vi "浊度电极校准.vi"() -> ()   [LabVIEW 2016, in "斯坦道多参数.lvlib"]
uses:
  <vilib>/Utility/miscctls.llb/LVPointTypeDef.ctl
  <vilib>/Utility/miscctls.llb/LVPositionTypeDef.ctl
  <vilib>/Analysis/NI_AALBase.lvlib
panel:
  out "温度":dbl format="%#.2f"
  out "通讯状态":string
  out "电极状态标志":u16(ring) items=["OK"=0, "第一点校正通过"=1, "第二点校正通过"=2, "悬浮物两点校准第一点校正通过"=11, "悬浮物两点校准第二点校正通过"=12, "浊度三点校正第一点校正通过"=31, "浊度三点校正第二点校正通过"=32, "浊度三点校正第三点校正通过"=33]
  out "第三点校准值":dbl
  out "标液3":dbl
  out "第二点校准值":dbl
  out "第一点校准值":dbl
  in  "校准停止":bool
  in  "校准启动":bool
  in  "校准模式":enum16{"两点校准", "单点校准", "三点校准"}(ring)
  out "最小值":sgl format="%#.2f"
  out "最大值":sgl format="%#.2f"
  out "波形图表":sgl(graph) caption="历史曲线"
  out "mean":dbl caption="均值" format="%#.2f"
  out "standard deviation":dbl caption="标准差" format="%#.2f"
  out "变异系数":dbl format="%#.6f"
  out "测量值":dbl format="%#.2f"
  out "提示":string
  out "标液2":dbl
  out "标液1":dbl
  out "原始读取值":dbl caption="信号值" format="%#.2f"
  out "偏移值补偿":dbl format="%#.2f"
  out "电极斜率":dbl format="%#.6f"
  out "电极零点":dbl format="%#.6f"
  # "浊度电极设定"
  # "℃"
  # "NTU"
  # "%"
  # "NTU"
  # "请选择校准模式:"
  # "NTU"
  # "NTU"
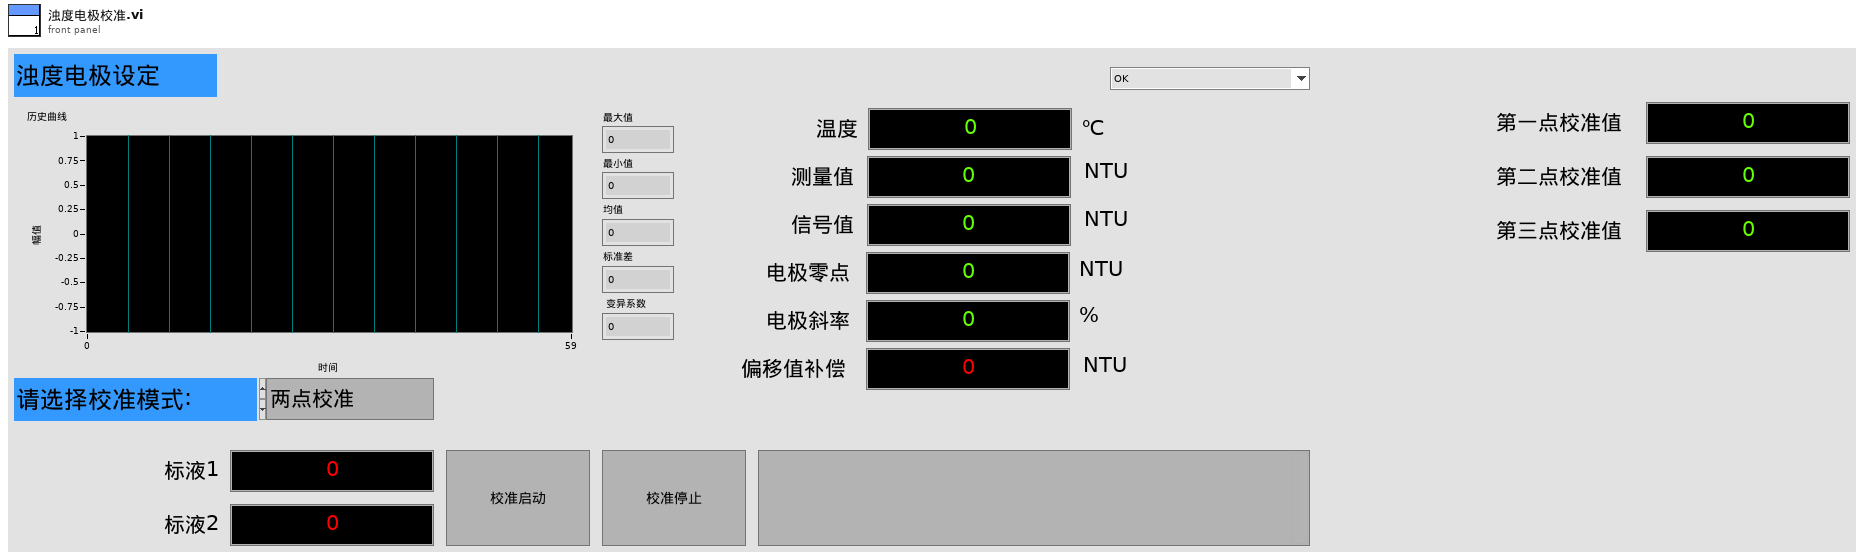
[diagram p1: front panel]
types:
  T1 = typedef "LVPointTypeDef.ctl" = cluster{"Horizontal":i16, "Vertical":i16}
  T2 = typedef "斯坦道多参数.lvlib/校准步骤.ctl" = enum16{"待机", "放置第一点标液", "第一点校准启动", "第一点校准写入", "第一点校准失败", "放置第二点标液", "第二点校准启动", "第二点校准写入", "第二点校准失败", "放置第三点标液", "第三点校准启动", "第三点校准写入", "第三点校准失败", "校准结果写入", "校准结束"}
  T3 = cluster{"电极状态标志":u16, "电极型号标志":u16, "浊度测量值":sgl, "温度测量值":sgl, "浊度信号值":sgl, "浊度偏移修正值":sgl, "温度偏移修正值":sgl, "手动温度补偿值":sgl, "浊度电极零点":sgl, "浊度电极斜率":sgl, "第1点标准值记录":sgl, "第1点信号值记录":sgl, "第1点温度值记录":sgl, "第2点标准值记录":sgl, "第2点信号值记录":sgl, "第2点温度值记录":sgl, "命令滤波设定":u16, "温度模式":enum16{"ATC", "MTC"}, "生产批次":u16, "电极序号":u16, "串口地址":u16, "串口波特率":enum16{"9600", "19200", "115200"}, "串口校验位":enum16{"NONE", "ODD", "EVEN"}, "串口停止位":enum16{"1bit", "2bit"}, "第一点标准值":sgl, "第二点标准值":sgl, "第三点标准值":sgl}
  T4 = typedef "LVPositionTypeDef.ctl" = cluster{"Left":i32, "Top":i32}
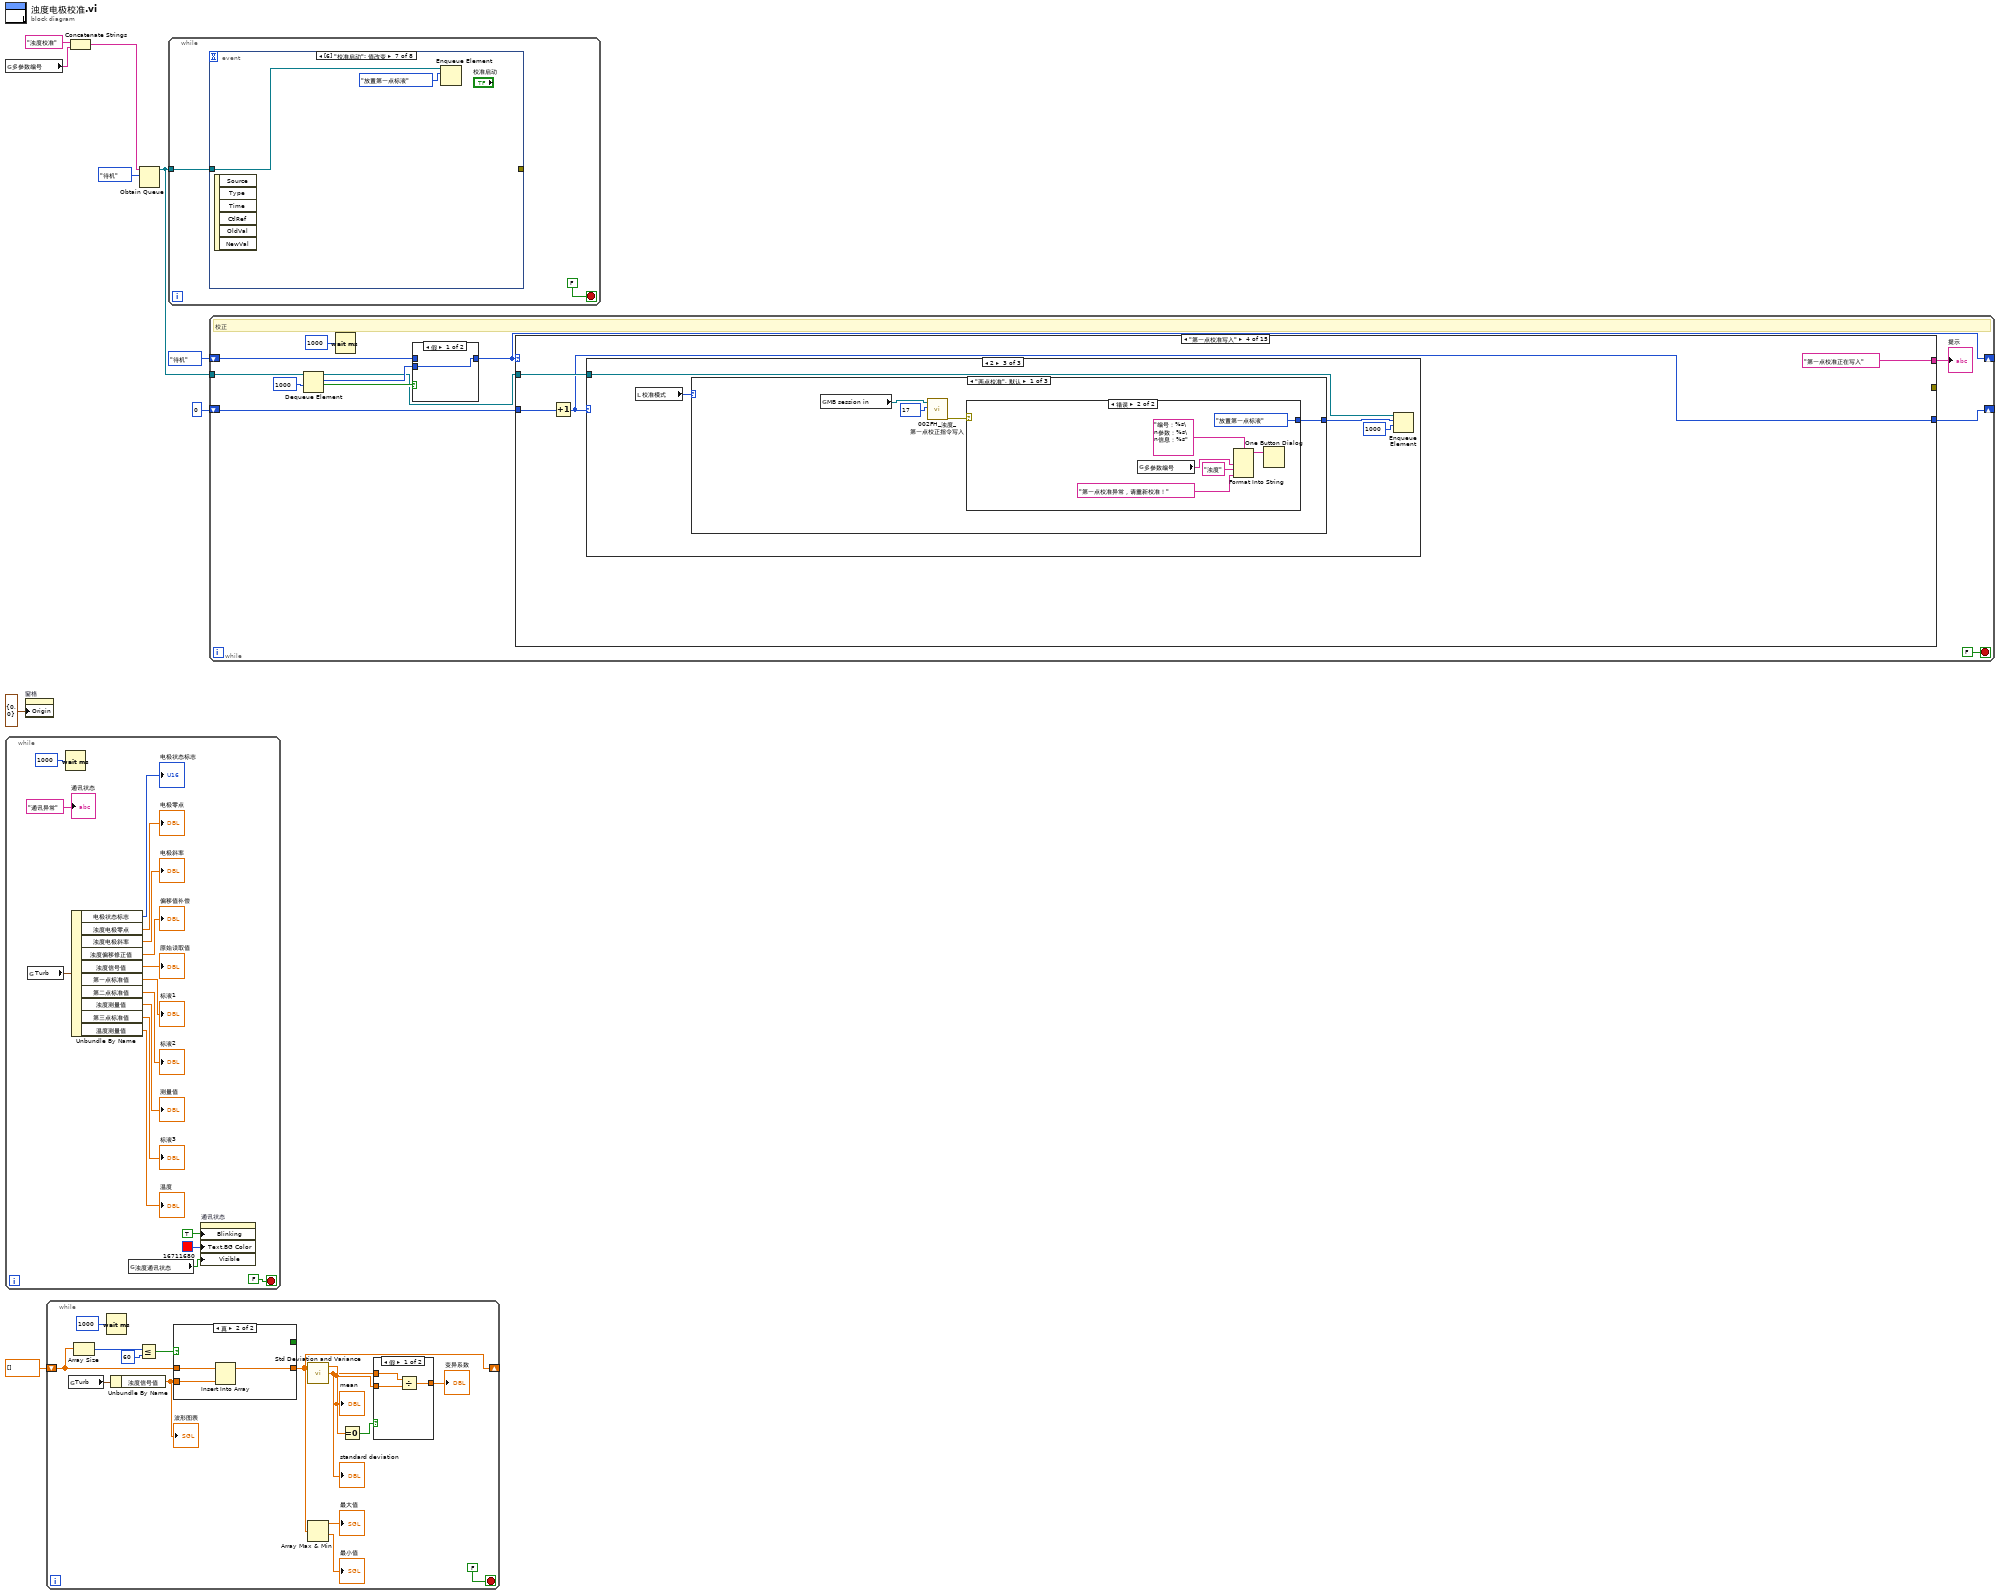
[diagram p0: block diagram]
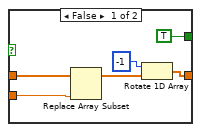
[diagram p3: hidden frame]
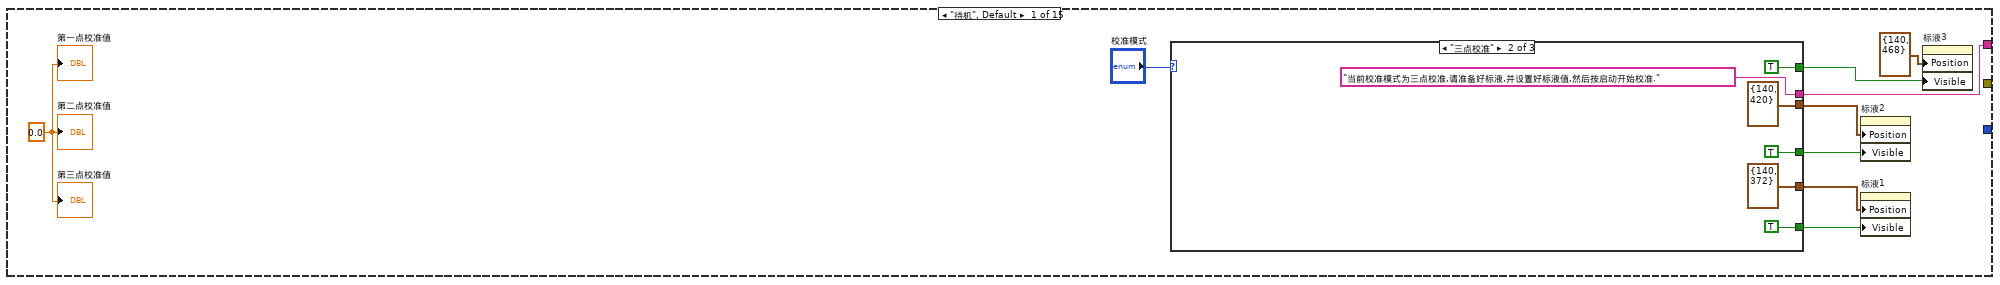
[diagram p5: hidden frame]
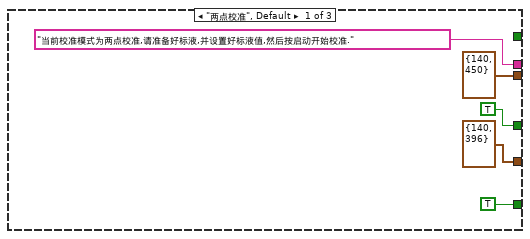
[diagram p6: hidden frame]
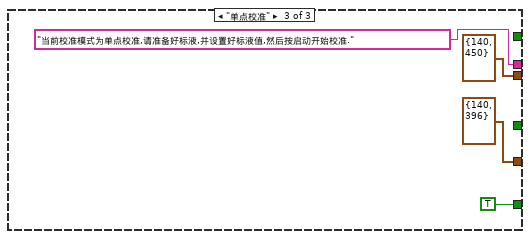
[diagram p7: hidden frame]
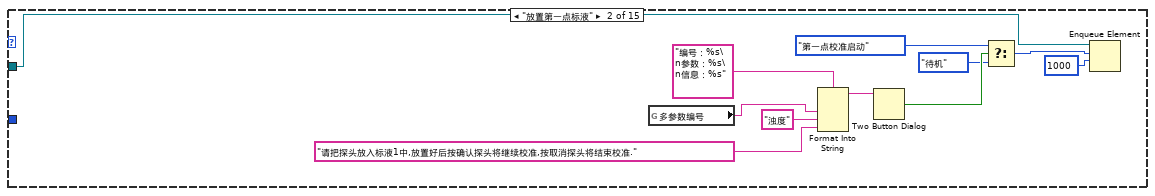
[diagram p8: hidden frame]
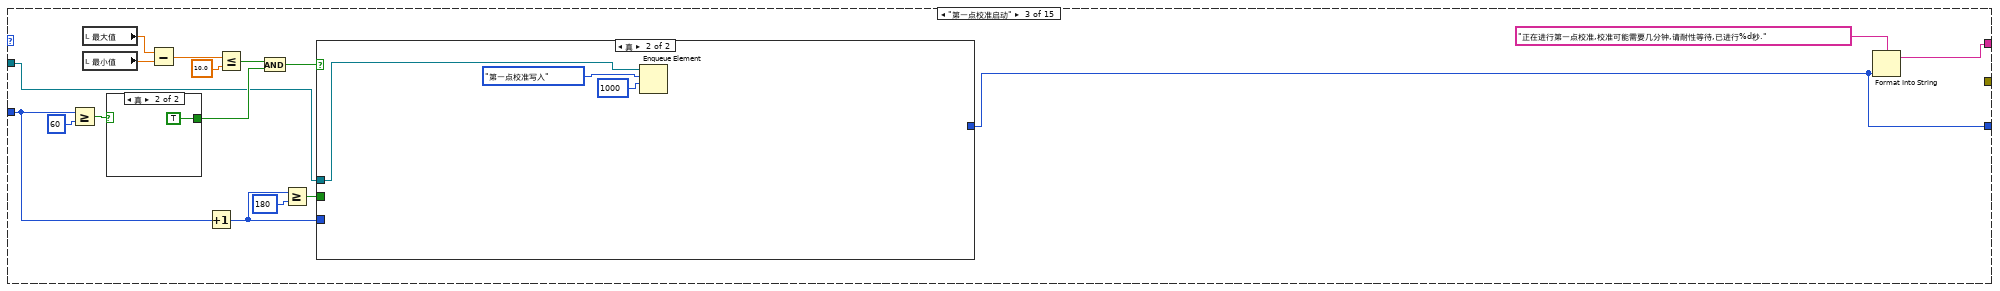
[diagram p9: hidden frame]
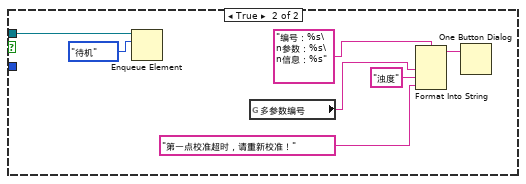
[diagram p11: hidden frame]
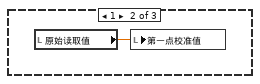
[diagram p14: hidden frame]
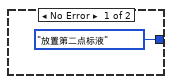
[diagram p15: hidden frame]
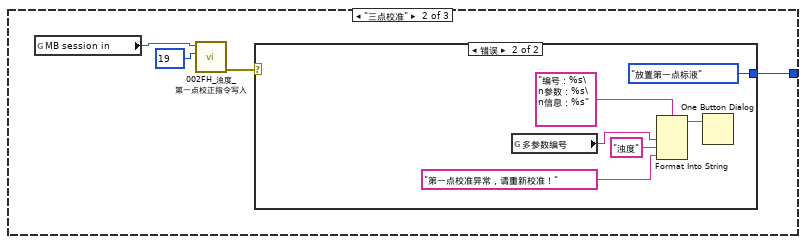
[diagram p16: hidden frame]
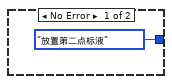
[diagram p17: hidden frame]
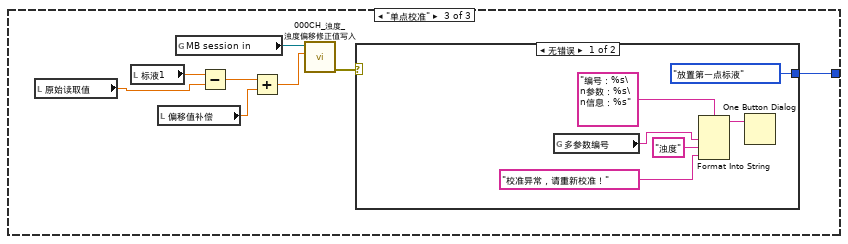
[diagram p18: hidden frame]
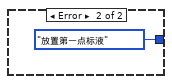
[diagram p19: hidden frame]
diagram:
  n1 = global read "多参数全局变量.vi" "多参数编号"() -> (w1:string)
  n2 = while {
    stop <- FALSE stop-if-true
    n3 = global read "国弘过程全局变量.vi" "Turb"() -> (w24:T3)
    n4 = Wait (ms)(milliseconds to wait=u32 1000 ("等待时间（毫秒）")) -> ()  [unwired: 1 out]
    n5 = Unbundle By Name(w24) -> ("电极状态标志"=→"电极状态标志":u16, "浊度电极零点"=→"电极零点":sgl, "浊度电极斜率"=→"电极斜率":sgl, "浊度偏移修正值"=→"偏移值补偿":sgl, "浊度信号值"=→"原始读取值":sgl, "第一点标准值"=→"标液1":sgl, "第二点标准值"=→"标液2":sgl, "浊度测量值"=→"测量值":sgl, "第三点标准值"=→"标液3":sgl, "温度测量值"=→"温度":sgl)
    n6 = global read "多参数全局变量.vi" "浊度通讯状态"() -> (w12:bool)
    n7 = property on="通讯状态" class="Str"("Blinking"=TRUE ("闪烁"), "Text.BG Color"=u32 16711680, "Visible"=w12) -> ()  [unwired: 2 in, 2 out]
    "通讯状态" <- "通讯异常" ("当前串口")
  }
  n8 = property on="窗格" class="Pane"("Origin"=T1 {"Horizontal"=0, "Vertical"=0} ("原点")) -> ()  [unwired: 2 in, 2 out]
  n9 = while {
    shift-right: [w30] -> _
    shift-left: sgl[] [] -> [w37]
    stop <- FALSE stop-if-true
    n10 = global read "国弘过程全局变量.vi" "Turb"() -> (w31:T3)
    n11 = Array Size(array=w37) -> (size(s)=w39:i32)
    n12 = Wait (ms)(milliseconds to wait=u32 1000 ("等待时间（毫秒）")) -> ()  [unwired: 1 out]
    n13 = Unbundle By Name(w31) -> ("浊度信号值"=w27:sgl)
    "波形图表" <- w27
    n14 = Less Or Equal?(x=w39, y=60) -> (x <= y?=w38:bool)
    n15 = case shown="真" w38 {
      tunnel: w37 -> [w50 w53]
      tunnel: w27 -> [w48 w52]
      tunnel: [w46 w51] -> w30
      tunnel: [TRUE _] -> _
      frame False {
        n16 = Replace Array Subset(array=w50, new element=w48) -> (w49:sgl[])  [unwired: 1 in]
        n17 = Rotate 1D Array(1:w49, 2:-1 ("n")) -> (0:w46:sgl[])
      }
      frame True {
        n18 = Insert Into Array(array=w53, new element=w52) -> (w51:sgl[])  [unwired: 1 in]
      }
    }
    n19 = call <vilib>:"Std Deviation and Variance.vi"("X"=w30) -> ("mean"=w35:dbl, "standard deviation"=w34:dbl)  [unwired: 1 in, 1 out]
    "mean" <- w35
    "standard deviation" <- w34
    n20 = Array Max & Min(array=w30) -> (max value=→"最大值":sgl, min value=→"最小值":sgl)  [unwired: 2 out]
    n21 = Equal To 0?(x=w35) -> (x = 0?=w36:bool)
    n22 = case shown="假" w36 {
      tunnel: w34 -> [w44 _]
      tunnel: [w43 _] -> w33
      tunnel: w35 -> [w42 _]
      frame False {
        n23 = Divide(x=w44, y=w42) -> (x/y=w43:dbl)
      }
      frame True {
      }
    }
    "变异系数" <- w33
  }
  n24 = Concatenate Strings("浊度校准" ("名称（未命名）"), w1) -> (w2:string)
  n25 = Obtain Queue(name (unnamed)=w2, element data type=校准步骤."待机" ("枚举")) -> (queue out=w4:refnum<queue>)  [unwired: 3 in, 2 out]
  n26 = while {
    tunnel: w4 -> [w54]
    stop <- FALSE stop-if-true
    n27 = event shown="[6] \"校准启动\": 值改变" {
      selector: _ -> [_ _ _ _ _ _ _ _]
      dyn-events: _ -> [_ _ _ _ _ _ _ _]
      timeout: _ -> [_ _ _ _ _ _ _ _]
      tunnel: [_ _ w61 w64 w68 w71 _ _] -> _
      tunnel: w54 -> [_ _ _ _ _ _ w72 w74]
      event Timeout {
        n28 = event-data() -> ()  [unwired: 1 in, 3 out]
      }
      event "偏移值补偿", "标液1", "标液2", "标液3": Mouse Down {
        n29 = event-data() -> ("CtlRef"=w56:refnum<vi>)  [unwired: 1 in, 7 out]
        n30 = property class="DigNum (严格)"(reference=w56) -> (reference out=w57:refnum<vi>, "Value"=w58:dbl)  [unwired: 1 in, 1 out]
        n31 = call "数字键盘.vi"("OldNumber"=w58) -> ("NewNumber"=w59:dbl)  [unwired: 1 in]
        n32 = property class="DigNum (严格)"(reference=w57, "Val(Sgnl)"=w59) -> ()  [unwired: 1 in, 2 out]
      }
      event "偏移值补偿": Value Change {
        n33 = event-data() -> ("NewVal"=w62:dbl)  [unwired: 1 in, 5 out]
        n34 = global read "多参数全局变量.vi" "MB session in"() -> (w60:refnum<class "MB_Master.lvclass">)
        n35 = call "000CH_浊度_浊度偏移修正值写入.vi"("数值"=w62, "MB session in"=w60) -> ("error out"=w61:errorcluster)  [unwired: 8 in, 1 out]
      }
      event "标液1": Value Change {
        n36 = event-data() -> ("NewVal"=w65:dbl)  [unwired: 1 in, 5 out]
        n37 = global read "多参数全局变量.vi" "MB session in"() -> (w63:refnum<class "MB_Master.lvclass">)
        n38 = call "0030H_浊度_第一点标准值写入.vi"("数值"=w65, "MB session in"=w63) -> ("error out"=w64:errorcluster)  [unwired: 8 in, 1 out]
      }
      event "标液2": Value Change {
        n39 = event-data() -> ("NewVal"=w67:dbl)  [unwired: 1 in, 5 out]
        n40 = global read "多参数全局变量.vi" "MB session in"() -> (w66:refnum<class "MB_Master.lvclass">)
        n41 = call "0033H_浊度_第二点标准值写入.vi"("数值"=w67, "MB session in"=w66) -> ("error out"=w68:errorcluster)  [unwired: 8 in, 1 out]
      }
      event "标液3": Value Change {
        n42 = event-data() -> ("NewVal"=w70:dbl)  [unwired: 1 in, 5 out]
        n43 = global read "多参数全局变量.vi" "MB session in"() -> (w69:refnum<class "MB_Master.lvclass">)
        n44 = call "0036H_浊度_第三点标准值写入.vi"("数值"=w70, "MB session in"=w69) -> ("error out"=w71:errorcluster)  [unwired: 8 in, 1 out]
      }
      event "校准启动": Value Change {
        n45 = event-data() -> ()  [unwired: 1 in, 6 out]
        n46 = Enqueue Element(queue=w72, element=校准步骤."放置第一点标液" ("元素")) -> ()  [unwired: 2 in, 3 out]
      }
      event "校准停止": Value Change {
        n47 = event-data() -> ()  [unwired: 1 in, 6 out]
        n48 = Flush Queue(queue=w74) -> (queue out=w75:refnum<queue>)  [unwired: 1 in, 2 out]
        n49 = Enqueue Element(queue=w75, element=校准步骤."待机" ("元素"), timeout in ms (-1)=1000 ("超时毫秒(-1)")) -> ()  [unwired: 1 in, 3 out]
      }
    }
  }
  n50 = while "While循环" {
    shift-right: [w79] -> _
    shift-left: 校准步骤."待机" ("枚举") -> [w81]
    shift-right: [w78] -> _
    shift-left: 0 -> [w87]
    tunnel: w4 -> [w82]
    stop <- FALSE stop-if-true
    # "校正"
    n51 = Dequeue Element(queue=w82, timeout in ms (-1)=1000 ("超时毫秒(-1)")) -> (queue out=w80:refnum<queue>, element=w83:T2, timed out?=w84:bool)  [unwired: 1 in, 1 out]
    n52 = Wait (ms)(milliseconds to wait=u32 1000 ("等待时间（毫秒）")) -> ()  [unwired: 1 out]
    n53 = case shown="假" w84 {
      tunnel: w83 -> [w90 _]
      tunnel: [w90 w91] -> w79
      tunnel: w81 -> [_ w91]
      frame False {
      }
      frame True {
      }
    }
    n54 = case shown="\"第一点校准写入\"" w79 {
      tunnel: [w99 _ w128 "第一点校准正在写入" ("提示") _ _ w219 "第二点校准正在写入" ("提示") "第二点校准失败" ("提示") _ "第三点校准正在写入" ("提示") w315 "第三点校准失败" ("提示") w349 w384] -> w86
      tunnel: w87 -> [_ _ w129 w162 _ _ w220 w252 _ _ w297 w316 _ _ _]
      tunnel: [_ _ w127 w160 _ _ w218 w250 _ _ w295 w314 _ _ _] -> w78
      tunnel: w80 -> [_ w121 w130 w161 _ w211 w221 w251 _ w289 w296 w317 _ w355 _]
      tunnel: [_ _ _ _ _ _ _ _ _ _ _ _ _ w354 _] -> _
      frame "待机", Default {
        w92 = 0.0 ("第一点校准值")
        n55 = case shown="\"三点校准\"" "校准模式" {
          tunnel: ["当前校准模式为两点校准,请准备好标液,并设置好标液值,然后按启动开始校准." ("提示") "当前校准模式为三点校准,请准备好标液,并设置好标液值,然后按启动开始校准." ("提示") "当前校准模式为单点校准,请准备好标液,并设置好标液值,然后按启动开始校准." ("提示")] -> w99
          tunnel: [TRUE ("可见") TRUE ("可见") _] -> w95
          tunnel: [T4 {"Left"=140, "Top"=396} ("位置") T4 {"Left"=140, "Top"=372} ("位置") T4 {"Left"=140, "Top"=396} ("位置")] -> w98
          tunnel: [T4 {"Left"=140, "Top"=450} ("位置 2") T4 {"Left"=140, "Top"=420} ("位置 2") T4 {"Left"=140, "Top"=450} ("位置 2")] -> w97
          tunnel: [_ TRUE ("可见") _] -> w94
          tunnel: [TRUE ("可见") TRUE ("可见") TRUE ("可见")] -> w93
          frame "两点校准", Default {
          }
          frame "三点校准" {
          }
          frame "单点校准" {
          }
        }
        n56 = property on="标液2" class="DigNum (严格)"("Position"=w97, "Visible"=w95) -> ()  [unwired: 2 in, 2 out]
        n57 = property on="标液1" class="DigNum (严格)"("Position"=w98, "Visible"=w93) -> ()  [unwired: 2 in, 2 out]
        n58 = property on="标液3" class="DigNum (严格)"("Position"=T4 {"Left"=140, "Top"=468} ("位置 3"), "Visible"=w94) -> ()  [unwired: 2 in, 2 out]
        "第一点校准值" <- w92
        "第二点校准值" <- w92
        "第三点校准值" <- w92
      }
      frame "放置第一点标液" {
        n59 = global read "多参数全局变量.vi" "多参数编号"() -> (w119:string)
        n60 = Format Into String(format string="编号：%s\n参数：%s\n信息：%s" ("格式字符串"), w119, "浊度" ("输入 2"), "请把探头放入标液1中,放置好后按确认探头将继续校准,按取消探头将结束校准." ("消息")) -> (resulting string=w116:string)  [unwired: 2 in, 1 out]
        n61 = Two Button Dialog(message=w116) -> (T button?=w125:bool)  [unwired: 2 in]
        n62 = Select(t=校准步骤."第一点校准启动" ("元素"), s=w125, f=校准步骤."待机" ("元素")) -> (s? t:f=w122:T2)
        n63 = Enqueue Element(queue=w121, element=w122, timeout in ms (-1)=1000 ("超时毫秒(-1)")) -> ()  [unwired: 1 in, 3 out]
      }
      frame "第一点校准启动" {
        n64 = Greater Or Equal?(x=w129, y=60) -> (x >= y?=w136:bool)
        n65 = local read "最大值"() -> (w139:sgl)
        n66 = local read "最小值"() -> (w138:sgl)
        n67 = case shown="真" w136 {
          tunnel: [_ TRUE] -> w137
          frame False {
          }
          frame True {
          }
        }
        n68 = Subtract(x=w139, y=w138) -> (x-y=w140:sgl)
        n69 = Increment(x=w129) -> (x+1=w143:i32)
        n70 = Less Or Equal?(x=w140, y=10.0) -> (x <= y?=w133:bool)
        n71 = And(x=w133, y=w137) -> (x .and. y?=w141:bool)
        n72 = Greater Or Equal?(x=w143, y=180) -> (x >= y?=w142:bool)
        n73 = case shown="真" w141 {
          tunnel: w130 -> [w146 w158]
          tunnel: w142 -> [w147 _]
          tunnel: w143 -> [w145 _]
          tunnel: [w144 _] -> w127
          frame False {
            n74 = case shown="假" w147 {
              tunnel: w146 -> [_ w155]
              tunnel: w145 -> [w148 _]
              tunnel: [w148 _] -> w144
              frame False {
              }
              frame True {
                n75 = Enqueue Element(queue=w155, element=校准步骤."待机" ("元素")) -> ()  [unwired: 2 in, 3 out]
                n76 = global read "多参数全局变量.vi" "多参数编号"() -> (w152:string)
                n77 = Format Into String(format string="编号：%s\n参数：%s\n信息：%s" ("格式字符串"), w152, "浊度" ("输入 2"), "第一点校准超时，请重新校准！" ("error source (\" \")")) -> (resulting string=w150:string)  [unwired: 2 in, 1 out]
                n78 = One Button Dialog(message=w150) -> ()  [unwired: 1 in, 1 out]
              }
            }
          }
          frame True {
            n79 = Enqueue Element(queue=w158, element=校准步骤."第一点校准写入" ("元素"), timeout in ms (-1)=1000 ("超时毫秒(-1)")) -> ()  [unwired: 1 in, 3 out]
          }
        }
        n80 = Format Into String(format string="正在进行第一点校准,校准可能需要几分钟,请耐性等待,已进行%d秒." ("格式字符串"), w127) -> (resulting string=w128:string)  [unwired: 2 in, 1 out]
      }
      frame "第一点校准写入" {
        n81 = Increment(x=w162) -> (x+1=w160:i32)
        n82 = case shown="2" w160 {
          tunnel: w161 -> [_ _ w168]
          frame 0, Default {
          }
          frame 1 {
            n83 = local read "原始读取值"() -> (w164:dbl)
            n84 = local write "第一点校准值"(w164) -> ()
          }
          frame 2 {
            n85 = local read "校准模式"() -> (w167:enum16{"两点校准", "单点校准", "三点校准"})
            n86 = case shown="\"两点校准\", 默认" w167 {
              tunnel: [w169 w180 w193] -> w166
              frame "两点校准", Default {
                n87 = global read "多参数全局变量.vi" "MB session in"() -> (w172:refnum<class "MB_Master.lvclass">)
                n88 = call "002FH_浊度_第一点校正指令写入.vi"("数值"=u16 17, "MB session in"=w172) -> ("error out"=w170:errorcluster)  [unwired: 8 in, 1 out]
                n89 = case shown="错误" w170 {
                  tunnel: [校准步骤."放置第二点标液" ("元素") 校准步骤."放置第一点标液" ("元素")] -> w169
                  frame No Error {
                  }
                  frame Error {
                    n90 = global read "多参数全局变量.vi" "多参数编号"() -> (w178:string)
                    n91 = Format Into String(format string="编号：%s\n参数：%s\n信息：%s" ("格式字符串"), w178, "浊度" ("输入 2"), "第一点校准异常，请重新校准！" ("error source (\" \")")) -> (resulting string=w177:string)  [unwired: 2 in, 1 out]
                    n92 = One Button Dialog(message=w177) -> ()  [unwired: 1 in, 1 out]
                  }
                }
              }
              frame "三点校准" {
                n93 = global read "多参数全局变量.vi" "MB session in"() -> (w183:refnum<class "MB_Master.lvclass">)
                n94 = call "002FH_浊度_第一点校正指令写入.vi"("数值"=u16 19, "MB session in"=w183) -> ("error out"=w181:errorcluster)  [unwired: 8 in, 1 out]
                n95 = case shown="错误" w181 {
                  tunnel: [校准步骤."放置第二点标液" ("元素") 校准步骤."放置第一点标液" ("元素")] -> w180
                  frame No Error {
                  }
                  frame Error {
                    n96 = global read "多参数全局变量.vi" "多参数编号"() -> (w189:string)
                    n97 = Format Into String(format string="编号：%s\n参数：%s\n信息：%s" ("格式字符串"), w189, "浊度" ("输入 2"), "第一点校准异常，请重新校准！" ("error source (\" \")")) -> (resulting string=w188:string)  [unwired: 2 in, 1 out]
                    n98 = One Button Dialog(message=w188) -> ()  [unwired: 1 in, 1 out]
                  }
                }
              }
              frame "单点校准" {
                n99 = local read "原始读取值"() -> (w198:dbl)
                n100 = local read "标液1"() -> (w197:dbl)
                n101 = local read "偏移值补偿"() -> (w191:dbl)
                n102 = global read "多参数全局变量.vi" "MB session in"() -> (w196:refnum<class "MB_Master.lvclass">)
                n103 = Subtract(x=w197, y=w198) -> (x-y=w195:dbl)
                n104 = Add(x=w195, y=w191) -> (x+y=w192:dbl)
                n105 = call "000CH_浊度_浊度偏移修正值写入.vi"("数值"=w192, "MB session in"=w196) -> ("error out"=w194:errorcluster)  [unwired: 8 in, 1 out]
                n106 = case shown="无错误" w194 {
                  tunnel: [校准步骤."放置第一点标液" ("元素") 校准步骤."放置第一点标液" ("元素")] -> w193
                  frame No Error {
                    n107 = global read "多参数全局变量.vi" "多参数编号"() -> (w201:string)
                    n108 = Format Into String(format string="编号：%s\n参数：%s\n信息：%s" ("格式字符串"), w201, "浊度" ("输入 2"), "校准异常，请重新校准！" ("error source (\" \")")) -> (resulting string=w202:string)  [unwired: 2 in, 1 out]
                    n109 = One Button Dialog(message=w202) -> ()  [unwired: 1 in, 1 out]
                  }
                  frame Error {
                  }
                }
              }
            }
            n110 = Enqueue Element(queue=w168, element=w166, timeout in ms (-1)=1000 ("超时毫秒(-1)")) -> ()  [unwired: 1 in, 3 out]
          }
        }
      }
      frame "第一点校准失败" {
      }
      frame "放置第二点标液" {
        n111 = global read "多参数全局变量.vi" "多参数编号"() -> (w209:string)
        n112 = Format Into String(format string="编号：%s\n参数：%s\n信息：%s" ("格式字符串"), w209, "浊度" ("输入 2"), "请把探头放入标液2中,放置好后按确认探头将继续校准,按取消探头将结束校准." ("消息")) -> (resulting string=w206:string)  [unwired: 2 in, 1 out]
        n113 = Two Button Dialog(message=w206) -> (T button?=w215:bool)  [unwired: 2 in]
        n114 = Select(t=校准步骤."第二点校准启动" ("元素"), s=w215, f=校准步骤."待机" ("元素")) -> (s? t:f=w212:T2)
        n115 = Enqueue Element(queue=w211, element=w212, timeout in ms (-1)=1000 ("超时毫秒(-1)")) -> ()  [unwired: 1 in, 3 out]
      }
      frame "第二点校准启动" {
        n116 = Greater Or Equal?(x=w220, y=60) -> (x >= y?=w226:bool)
        n117 = local read "最大值"() -> (w229:sgl)
        n118 = local read "最小值"() -> (w228:sgl)
        n119 = case shown="真" w226 {
          tunnel: [_ TRUE] -> w227
          frame False {
          }
          frame True {
          }
        }
        n120 = Subtract(x=w229, y=w228) -> (x-y=w230:sgl)
        n121 = Increment(x=w220) -> (x+1=w233:i32)
        n122 = Less Or Equal?(x=w230, y=10.0) -> (x <= y?=w223:bool)
        n123 = And(x=w223, y=w227) -> (x .and. y?=w231:bool)
        n124 = Greater Or Equal?(x=w233, y=180) -> (x >= y?=w232:bool)
        n125 = case shown="假" w231 {
          tunnel: w221 -> [w236 w248]
          tunnel: w232 -> [w237 _]
          tunnel: w233 -> [w235 _]
          tunnel: [w234 _] -> w218
          frame False {
            n126 = case shown="真" w237 {
              tunnel: w236 -> [_ w245]
              tunnel: w235 -> [w238 _]
              tunnel: [w238 _] -> w234
              frame False {
              }
              frame True {
                n127 = Enqueue Element(queue=w245, element=校准步骤."放置第二点标液" ("元素")) -> ()  [unwired: 2 in, 3 out]
                n128 = global read "多参数全局变量.vi" "多参数编号"() -> (w242:string)
                n129 = Format Into String(format string="编号：%s\n参数：%s\n信息：%s" ("格式字符串"), w242, "浊度" ("输入 2"), "第二点校准超时，请重新校准！" ("error source (\" \")")) -> (resulting string=w240:string)  [unwired: 2 in, 1 out]
                n130 = One Button Dialog(message=w240) -> ()  [unwired: 1 in, 1 out]
              }
            }
          }
          frame True {
            n131 = Enqueue Element(queue=w248, element=校准步骤."第二点校准写入" ("元素"), timeout in ms (-1)=1000 ("超时毫秒(-1)")) -> ()  [unwired: 1 in, 3 out]
          }
        }
        n132 = Format Into String(format string="正在进行第二点校准,校准可能需要几分钟,请耐性等待,已进行%d秒." ("格式字符串"), w218) -> (resulting string=w219:string)  [unwired: 2 in, 1 out]
      }
      frame "第二点校准写入" {
        n133 = Increment(x=w252) -> (x+1=w250:i32)
        n134 = case shown="0, 默认" w250 {
          tunnel: w251 -> [_ _ w258]
          frame 0, Default {
          }
          frame 1 {
            n135 = local read "原始读取值"() -> (w254:dbl)
            n136 = local write "第二点校准值"(w254) -> ()
          }
          frame 2 {
            n137 = local read "校准模式"() -> (w255:enum16{"两点校准", "单点校准", "三点校准"})
            n138 = case shown="\"三点校准\"" w255 {
              tunnel: [w262 w273] -> w256
              frame "两点校准", Default {
                n139 = global read "多参数全局变量.vi" "MB session in"() -> (w259:refnum<class "MB_Master.lvclass">)
                n140 = call "0032H_浊度_第二点校正指令写入.vi"("数值"=u16 33, "MB session in"=w259) -> ("error out"=w260:errorcluster)  [unwired: 8 in, 1 out]
                n141 = case shown="错误" w260 {
                  tunnel: [校准步骤."校准结果写入" ("元素") 校准步骤."放置第二点标液" ("元素")] -> w262
                  frame No Error {
                  }
                  frame Error {
                    n142 = global read "多参数全局变量.vi" "多参数编号"() -> (w267:string)
                    n143 = Format Into String(format string="编号：%s\n参数：%s\n信息：%s" ("格式字符串"), w267, "浊度" ("输入 2"), "第二点校准异常，请重新校准！" ("error source (\" \")")) -> (resulting string=w266:string)  [unwired: 2 in, 1 out]
                    n144 = One Button Dialog(message=w266) -> ()  [unwired: 1 in, 1 out]
                  }
                }
              }
              frame "三点校准" {
                n145 = global read "多参数全局变量.vi" "MB session in"() -> (w270:refnum<class "MB_Master.lvclass">)
                n146 = call "0032H_浊度_第二点校正指令写入.vi"("数值"=u16 35, "MB session in"=w270) -> ("error out"=w271:errorcluster)  [unwired: 8 in, 1 out]
                n147 = case shown="错误" w271 {
                  tunnel: [校准步骤."放置第三点标液" ("元素") 校准步骤."放置第二点标液" ("元素")] -> w273
                  frame No Error {
                  }
                  frame Error {
                    n148 = global read "多参数全局变量.vi" "多参数编号"() -> (w278:string)
                    n149 = Format Into String(format string="编号：%s\n参数：%s\n信息：%s" ("格式字符串"), w278, "浊度" ("输入 2"), "第二点校准异常，请重新校准！" ("error source (\" \")")) -> (resulting string=w277:string)  [unwired: 2 in, 1 out]
                    n150 = One Button Dialog(message=w277) -> ()  [unwired: 1 in, 1 out]
                  }
                }
              }
            }
            n151 = Enqueue Element(queue=w258, element=w256, timeout in ms (-1)=1000 ("超时毫秒(-1)")) -> ()  [unwired: 1 in, 3 out]
          }
        }
      }
      frame "第二点校准失败" {
      }
      frame "放置第三点标液" {
        n152 = global read "多参数全局变量.vi" "多参数编号"() -> (w285:string)
        n153 = global read "多参数全局变量.vi" "多参数编号"() -> (w287:string)
        n154 = Format Into String(format string="编号：%s\n参数：%s\n信息：%s" ("格式字符串"), w285, "浊度" ("输入 2"), "请把探头放入标液3中,放置好后按确认探头将继续校准,按取消探头将结束校准." ("消息")) -> (resulting string=w282:string)  [unwired: 2 in, 1 out]
        n155 = Concatenate Strings(w287, w282) -> (w288:string)
        n156 = Two Button Dialog(message=w288) -> (T button?=w293:bool)  [unwired: 2 in]
        n157 = Select(t=校准步骤."第三点校准启动" ("元素"), s=w293, f=校准步骤."待机" ("元素")) -> (s? t:f=w290:T2)
        n158 = Enqueue Element(queue=w289, element=w290, timeout in ms (-1)=1000 ("超时毫秒(-1)")) -> ()  [unwired: 1 in, 3 out]
      }
      frame "第三点校准写入" {
        n159 = Increment(x=w297) -> (x+1=w295:i32)
        n160 = case shown="1" w295 {
          tunnel: w296 -> [_ _ w305]
          frame 0, Default {
          }
          frame 1 {
            n161 = local read "原始读取值"() -> (w299:dbl)
            n162 = local write "第二点校准值"(w299) -> ()
          }
          frame 2 {
            n163 = global read "多参数全局变量.vi" "MB session in"() -> (w300:refnum<class "MB_Master.lvclass">)
            n164 = call "0035H_浊度_第三点校正指令写入.vi"("数值"=u16 51, "MB session in"=w300) -> ("error out"=w301:errorcluster)  [unwired: 8 in, 1 out]
            n165 = case shown="错误" w301 {
              tunnel: [校准步骤."校准结果写入" ("元素") 校准步骤."放置第三点标液" ("元素")] -> w303
              frame No Error {
              }
              frame Error {
                n166 = global read "多参数全局变量.vi" "多参数编号"() -> (w310:string)
                n167 = Format Into String(format string="编号：%s\n参数：%s\n信息：%s" ("格式字符串"), w310, "浊度" ("输入 2"), "第三点校准异常，请重新校准！" ("error source (\" \")")) -> (resulting string=w309:string)  [unwired: 2 in, 1 out]
                n168 = One Button Dialog(message=w309) -> ()  [unwired: 1 in, 1 out]
              }
            }
            n169 = Enqueue Element(queue=w305, element=w303, timeout in ms (-1)=1000 ("超时毫秒(-1)")) -> ()  [unwired: 1 in, 3 out]
          }
        }
      }
      frame "第三点校准启动" {
        n170 = Greater Or Equal?(x=w316, y=60) -> (x >= y?=w322:bool)
        n171 = local read "最大值"() -> (w325:sgl)
        n172 = local read "最小值"() -> (w324:sgl)
        n173 = case shown="真" w322 {
          tunnel: [_ TRUE] -> w323
          frame False {
          }
          frame True {
          }
        }
        n174 = Subtract(x=w325, y=w324) -> (x-y=w326:sgl)
        n175 = Increment(x=w316) -> (x+1=w329:i32)
        n176 = Less Or Equal?(x=w326, y=10.0) -> (x <= y?=w319:bool)
        n177 = And(x=w319, y=w323) -> (x .and. y?=w327:bool)
        n178 = Greater Or Equal?(x=w329, y=180) -> (x >= y?=w328:bool)
        n179 = case shown="假" w327 {
          tunnel: w317 -> [w332 w344]
          tunnel: w328 -> [w333 _]
          tunnel: w329 -> [w331 _]
          tunnel: [w330 _] -> w314
          frame False {
            n180 = case shown="真" w333 {
              tunnel: w332 -> [_ w341]
              tunnel: w331 -> [w334 _]
              tunnel: [w334 _] -> w330
              frame False {
              }
              frame True {
                n181 = Enqueue Element(queue=w341, element=校准步骤."待机" ("元素")) -> ()  [unwired: 2 in, 3 out]
                n182 = global read "多参数全局变量.vi" "多参数编号"() -> (w338:string)
                n183 = Format Into String(format string="编号：%s\n参数：%s\n信息：%s" ("格式字符串"), w338, "浊度" ("输入 2"), "第三点校准超时，请重新校准！" ("error source (\" \")")) -> (resulting string=w336:string)  [unwired: 2 in, 1 out]
                n184 = One Button Dialog(message=w336) -> ()  [unwired: 1 in, 1 out]
              }
            }
          }
          frame True {
            n185 = Enqueue Element(queue=w344, element=校准步骤."第三点校准写入" ("元素"), timeout in ms (-1)=1000 ("超时毫秒(-1)")) -> ()  [unwired: 1 in, 3 out]
          }
        }
        n186 = Format Into String(format string="正在进行第三点校准,校准可能需要几分钟,请耐性等待,已进行%d秒." ("格式字符串"), w314) -> (resulting string=w315:string)  [unwired: 2 in, 1 out]
      }
      frame "第三点校准失败" {
      }
      frame "校准结果写入" {
        n187 = call "时间延迟"() -> ("error out"=w347:errorcluster)  [unwired: 11 in]
        n188 = Enqueue Element(queue=w355, element=校准步骤."校准结束" ("元素")) -> ()  [unwired: 2 in, 3 out]
        n189 = flat-sequence {
          tunnel: [w359] -> w350
          tunnel: w347 -> [_]
          frame #0 {
            n190 = global read "国弘过程全局变量.vi" "Turb"() -> (w358:T3)
            n191 = Unbundle By Name(w358) -> ("电极状态标志"=w357:u16)
            n192 = case shown="0, 默认" w357 {
              selector: w357 -> [_ w381]
              tunnel: [w360 w380] -> w359
              frame 0, Default {
                n193 = local read "校准模式"() -> (w361:enum16{"两点校准", "单点校准", "三点校准"})
                n194 = case shown="\"单点校准\"" w361 {
                  tunnel: [w367 w375 w379] -> w360
                  frame "两点校准", Default {
                    n195 = local read "第一点校准值"() -> (w365:dbl)
                    n196 = local read "第二点校准值"() -> (w363:dbl)
                    n197 = local read "标液1"() -> (w366:dbl)
                    n198 = local read "标液2"() -> (w362:dbl)
                    n199 = Format Into String(format string="校准结果：第一点校准值=%f，第一点标准值=%f,第二点校准值=%f，第二点标准值=%f." ("提示"), w365, w366, w363, w362) -> (resulting string=w367:string)  [unwired: 2 in, 1 out]
                  }
                  frame "三点校准" {
                    n200 = local read "第一点校准值"() -> (w373:dbl)
                    n201 = local read "第二点校准值"() -> (w372:dbl)
                    n202 = local read "第三点校准值"() -> (w369:dbl)
                    n203 = local read "标液1"() -> (w374:dbl)
                    n204 = local read "标液2"() -> (w370:dbl)
                    n205 = local read "标液3"() -> (w368:dbl)
                    n206 = Format Into String(format string="校准结果：第一点校准值=%f，第一点标准值=%f,第二点校准值=%f，第二点标准值=%f,第三点校准值=%f，第三点标准值=%f." ("提示"), w373, w374, w372, w370, w369, w368) -> (resulting string=w375:string)  [unwired: 2 in, 1 out]
                  }
                  frame "单点校准" {
                    n207 = local read "第一点校准值"() -> (w378:dbl)
                    n208 = local read "标液1"() -> (w376:dbl)
                    n209 = Format Into String(format string="校准结果：校准值=%f，标准值=%f。" ("提示"), w378, w376) -> (resulting string=w379:string)  [unwired: 2 in, 1 out]
                  }
                }
              }
              frame 3, 4 {
                n210 = case shown="3, 默认" w381 {
                  tunnel: ["校正失败，电极零点超出范围" "校正失败，电极斜率超出范围"] -> w380
                  frame 3, Default {
                  }
                  frame 4 {
                  }
                }
              }
            }
          }
        }
        n211 = global read "多参数全局变量.vi" "多参数编号"() -> (w352:string)
        n212 = Format Into String(format string="编号：%s\n参数：%s\n信息：%s" ("格式字符串"), w352, "浊度" ("输入 2"), w350) -> (resulting string=w349:string)  [unwired: 2 in, 1 out]
        n213 = One Button Dialog(message=w349) -> ()  [unwired: 1 in, 1 out]
        n214 = call "操作日志.vi"("table"="校准记录", "日志信息"=w349) -> ("error out"=w354:errorcluster)  [unwired: 9 in]
      }
      frame "校准结束" {
        n215 = local read "提示"() -> (w384:string)
      }
    }
    "提示" <- w86
  }
